vi "prueba-watchdog.vi"() -> ()   [LabVIEW 2015]
uses:
  <vilib>/RTwatchdog.llb/Watchdog expiration actions.ctl
panel:
  in  "milliseconds to wait":u32
  out "Numeric":i32
  in  "stop":bool
  out "error out 3":errorcluster
  out "error out 2":errorcluster
  out "error out":errorcluster
  in  "expiration actions":T1={"reset"=FALSE, "occurrence"=FALSE, "trigger protocol"=enum."active high", "trigger line"=enum."none", "disable watchdog on VI exit"=TRUE}
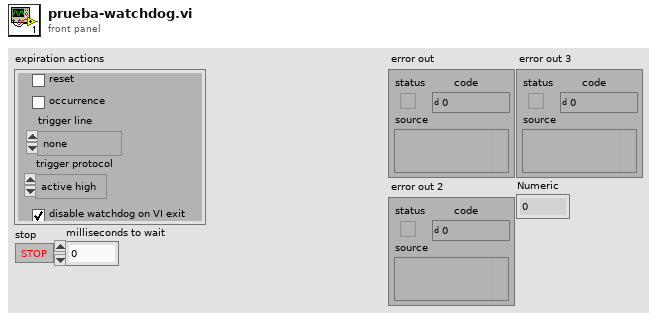
[diagram p1: front panel]
types:
  T1 = typedef "Watchdog expiration actions.ctl" = cluster{"reset":bool, "occurrence":bool, "trigger protocol":enum16{"active high", "active low", "open collector"}, "trigger line":enum16{"none", "line 0", "line 1", "line 2", "line 3", "line 4", "line 5", "line 6", "line 7", "SMB line 0"}, "disable watchdog on VI exit":bool}
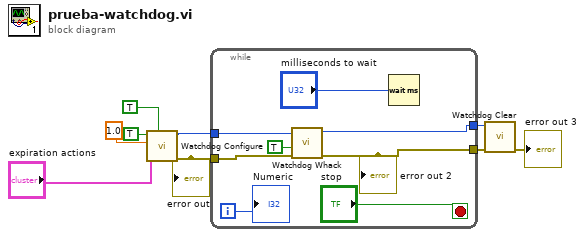
[diagram p0: block diagram]
diagram:
  n1 = call <vilib>:"Watchdog Configure.vi"("RESET"=TRUE, "expiration actions"="expiration actions", "timeout (1 sec)"=1.0, "DISABLE WDOG"=TRUE) -> ("error out"=w6:errorcluster, "watchdogID"=w8:u64)  [unwired: 2 in, 2 out]
  "error out" <- w6
  n2 = while {
    tunnel: w8 -> [w16]
    tunnel: [w15] -> w7
    tunnel: w6 -> [w14]
    tunnel: [w13] -> w5
    i -> [w11]
    stop <- "stop" stop-if-true
    n3 = call <vilib>:"Watchdog Whack.vi"("error in (no error)"=w14, "reset watchdog after expire? (F)"=TRUE, "watchdogID in"=w16) -> ("error out"=w13:errorcluster, "watchdogID out"=w15:u64)  [unwired: 2 in, 1 out]
    "error out 2" <- w13
    n4 = Wait (ms)(milliseconds to wait="milliseconds to wait") -> ()  [unwired: 1 out]
    "Numeric" <- w11
  }
  n5 = call <vilib>:"Watchdog Clear.vi"("error in (no error)"=w5, "watchdogID in"=w7) -> ("error out"=→"error out 3":errorcluster)  [unwired: 5 in]
